vi "Write Notification Msg Return Info.vi"(8 "Return Priority (Normal)":T1=enum."Normal", 9 "Topic Name":string, 10 "Message Enqueuer in":refnum<class "Message Enqueuer.lvclass">, 11 "Notification Msg":refnum<class "Notification Msg.lvclass">) -> (3 "Notification Msg Out":refnum<class "Notification Msg.lvclass">)   [LabVIEW 2015, in "Transport.lvlib" / "Notification Msg.lvclass"]
doc: "<License>\nCopyright © 2017 Composed Systems, LLC | All rights reserved\nwww.composed.io\n\nAuthor: Ethan Stern <ethan.stern@composed.io>\n\nThis software is provided \"AS IS\" WITHOUT WARRANTIES, either express or implied, AND IS FOR EDUCATIONAL PURPOSES ONLY.\n</License>"
uses:
  Notification Msg.lvclass
  <vilib>/ActorFramework/Message Enqueuer/Message Enqueuer.lvclass
  <vilib>/ActorFramework/Message Enqueuer/Message Priority.ctl
  Notification Msg.lvclass/Notification Msg.ctl
  AbstractMessages/PreAddressedMsg/PreAddressedMsg.lvclass/PreAddressedMsg.ctl
  AbstractMessages/PreAddressedMsg/PreAddressedMsg.lvclass
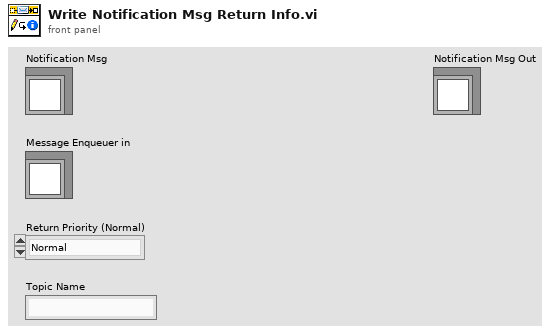
[diagram p1: front panel]
types:
  T1 = typedef "Actor Framework.lvlib/Message Enqueuer.lvclass/Message Priority.ctl" = enum16{"Low", "Normal", "High"}
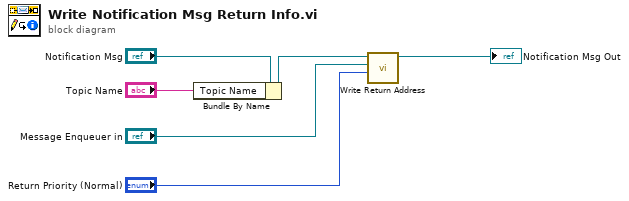
[diagram p0: block diagram]
diagram:
  n1 = Bundle By Name(cluster="Notification Msg", "Topic Name"="Topic Name") -> (w2:refnum<class "Notification Msg.lvclass">)
  n2 = call "Write Return Address.vi"("Return Priority (Normal)"="Return Priority (Normal)", "Return Address"="Message Enqueuer in", "PreAddressedMsg in"=w2) -> ("PreAddressedMsg out"=→"Notification Msg Out":refnum<class "Notification Msg.lvclass">)  [unwired: 8 in]
